vi "RGB to HSL.vi"(0 "RGB":u8[](array[numeric])) -> (4 "HSL":u8[](array[numeric]))   [LabVIEW 2016]
panel:
  out "Chroma":i16
  out "Min":i16
  out "Max":i16
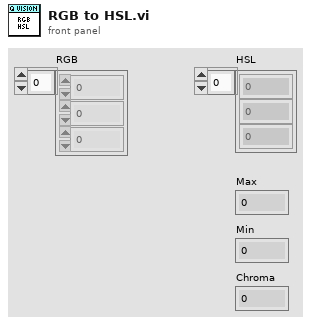
[diagram p1: front panel]
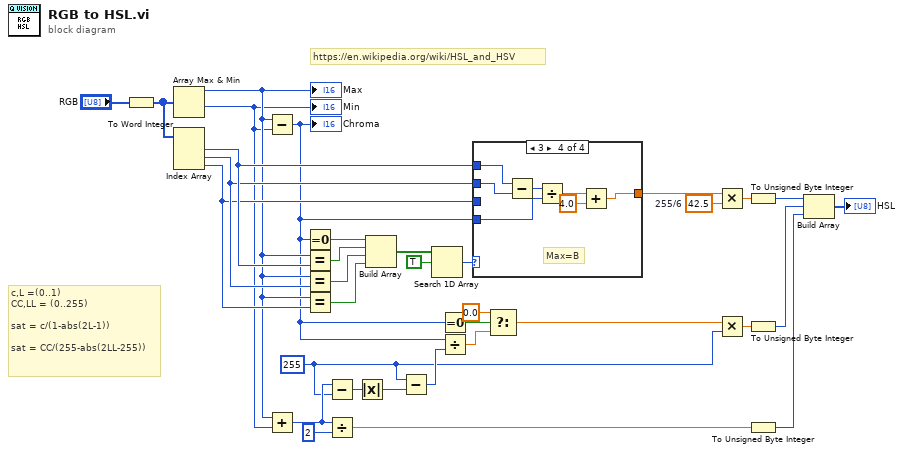
[diagram p0: block diagram]
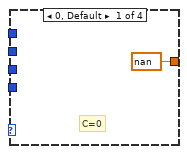
[diagram p2: hidden frame]
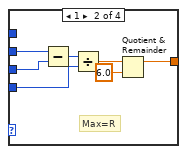
[diagram p3: hidden frame]
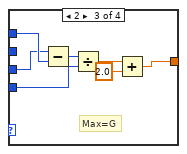
[diagram p4: hidden frame]
diagram:
  w1 = i16 255 ("y")
  w26 = 42.5  # 255/6
  # "c,L =(0..1)\nCC,LL = (0..255)\n\nsat = c/(1-abs(2L-1))\n\nsat = CC/(255-abs(2LL-255))"
  # "https://en.wikipedia.org/wiki/HSL_and_HSV"
  n1 = To Word Integer(number="RGB") -> (16bit integer=w7:i16[])
  n2 = Array Max & Min(array=w7) -> (max value=w6:i16, min value=w5:i16)  [unwired: 2 out]
  "Max" <- w6
  "Min" <- w5
  n3 = Index Array(array=w7) -> (element #1=w17:i16, element #2=w16:i16, element #3=w15:i16)  [unwired: 3 in]
  n4 = Subtract(x=w6, y=w5) -> (x-y=w4:i16)
  "Chroma" <- w4
  n5 = Add(x=w6, y=w5) -> (x+y=w3:i16)
  n6 = Equal To 0?(x=w4) -> (x = 0?=w34:bool)
  n7 = Equal?(x=w6, y=w17) -> (x = y?=w33:bool)
  n8 = Equal?(x=w6, y=w16) -> (x = y?=w32:bool)
  n9 = Equal?(x=w6, y=w15) -> (x = y?=w31:bool)
  n10 = Subtract(x=w3, y=w1) -> (x-y=w24:i16)
  n11 = Divide(x=w3, y=i16 2) -> (x/y=w12:dbl)
  n12 = Absolute Value(x=w24) -> (abs(x)=w23:i16)
  n13 = Build Array(w34, w33, w32, w31) -> (w30:bool[])
  n14 = Subtract(x=w1, y=w23) -> (x-y=w22:i16)
  n15 = Search 1D Array(1D array=w30, element=TRUE) -> (index of element=w28:i32)  [unwired: 1 in]
  n16 = Equal To 0?(x=w4) -> (x = 0?=w21:bool)
  n17 = Divide(x=w4, y=w22) -> (x/y=w20:dbl)
  n18 = case shown="3" w28 {
    tunnel: w4 -> [_ w39 w48 w55]
    tunnel: w17 -> [_ _ w47 w51]
    tunnel: w16 -> [_ w41 _ w50]
    tunnel: w15 -> [_ w40 w46 _]
    tunnel: [nan w36 w44 w53] -> w27
    frame 0, Default {
      # "C=0"
    }
    frame 1 {
      # "Max=R"
      n19 = Subtract(x=w41, y=w40) -> (x-y=w42:i16)
      n20 = Divide(x=w42, y=w39) -> (x/y=w38:dbl)
      n21 = Quotient & Remainder(x=w38, y=6.0) -> (x-y*floor(x/y)=w36:dbl)  [unwired: 1 out]
    }
    frame 2 {
      # "Max=G"
      n22 = Subtract(x=w46, y=w47) -> (x-y=w49:i16)
      n23 = Divide(x=w49, y=w48) -> (x/y=w45:dbl)
      n24 = Add(x=w45, y=2.0) -> (x+y=w44:dbl)
    }
    frame 3 {
      # "Max=B"
      n25 = Subtract(x=w51, y=w50) -> (x-y=w56:i16)
      n26 = Divide(x=w56, y=w55) -> (x/y=w54:dbl)
      n27 = Add(x=w54, y=4.0) -> (x+y=w53:dbl)
    }
  }
  n28 = Select(t=0.0, s=w21, f=w20) -> (s? t:f=w13:dbl)
  n29 = Multiply(x=w27, y=w26) -> (x*y=w14:dbl)
  n30 = Multiply(x=w13, y=w1) -> (x*y=w2:dbl)
  n31 = To Unsigned Byte Integer(number=w14) -> (unsigned 8bit integer=w11:u8)
  n32 = To Unsigned Byte Integer(number=w2) -> (unsigned 8bit integer=w10:u8)
  n33 = To Unsigned Byte Integer(number=w12) -> (unsigned 8bit integer=w9:u8)
  n34 = Build Array(w11, w10, w9) -> (→"HSL":u8[])
